vi "CALC arm angle.vi"() -> ()   [LabVIEW 2020]
uses:
  Robot Global Data.vi
panel:
  out "angle of arm pin to link pin":dbl
  out "length of arm pin to link":dbl
  in  "arm distance from center":dbl
  in  "adjust for PITCH?":bool=TRUE
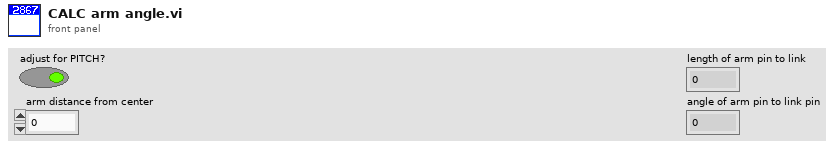
[diagram p1: front panel]
types:
  T1 = cluster{"gear ratio":cluster{"value":dbl, "descr":string}, "screw tpi":cluster{"value":dbl, "descr":string}, "shoulder AG":cluster{"value":dbl, "descr":string}, "shoulder to CTR":cluster{"value":dbl, "descr":string}, "shoulder to screw 0":cluster{"value":dbl, "descr":string}, "screw shuttle AG":cluster{"value":dbl, "descr":string}, "screw length":cluster{"value":dbl, "descr":string}, "screw to full front":cluster{"value":dbl, "descr":string}, "screw link":cluster{"value":dbl, "descr":string}, "lower arm length":cluster{"value":dbl, "descr":string}, "arm top":cluster{"value":dbl, "descr":string}, "shoulder to pin link Y":cluster{"value":dbl, "descr":string}, "shoulder to pin link X":cluster{"value":dbl, "descr":string}, "hook ht":cluster{"value":dbl, "descr":string}, "hook clear":cluster{"value":dbl, "descr":string}}
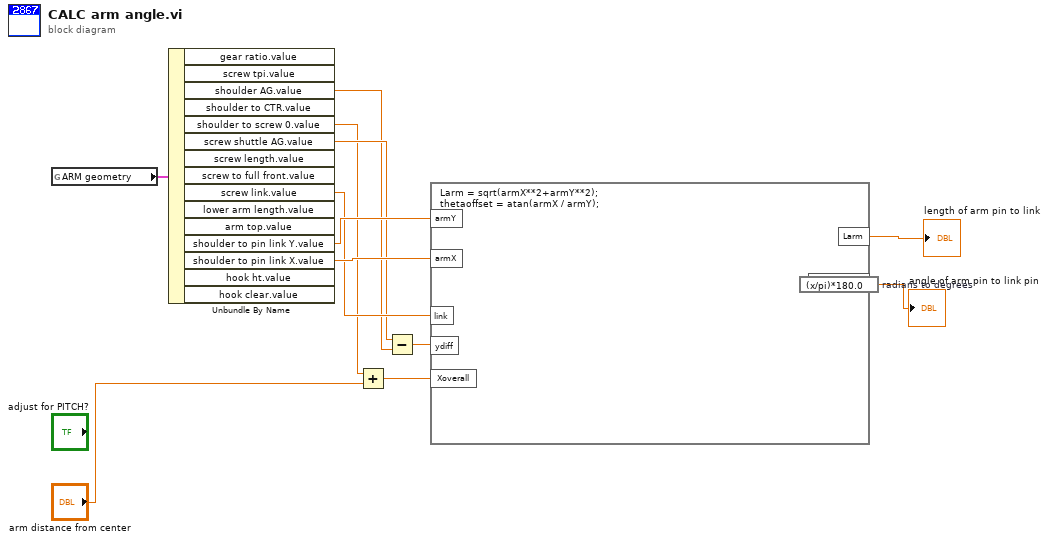
[diagram p0: block diagram]
diagram:
  n1 = global read "Robot Global Data.vi" "ARM geometry"() -> (w13:T1)
  n2 = Unbundle By Name(w13) -> ("shoulder AG.value"=w4:dbl, "shoulder to screw 0.value"=w1:dbl, "screw shuttle AG.value"=w5:dbl, "screw link.value"=w7:dbl, "shoulder to pin link Y.value"=w12:dbl, "shoulder to pin link X.value"=w11:dbl)  [unwired: 9 out]
  n3 = Add(x=w1, y="arm distance from center") -> (x+y=w3:dbl)
  n4 = Subtract(x=w5, y=w4) -> (x-y=w6:dbl)
  n5 = formula code="Larm = sqrt(armX**2+armY**2);\nthetaoffset = atan(armX / armY);"("armY"=w12, "armX"=w11, "link"=w7, "ydiff"=w6, "Xoverall"=w3) -> ("Larm"=→"length of arm pin to link":dbl, "thetaoffset"=w9:dbl)
  n6 = expression code="(x/pi)*180.0" "radians to degrees"(w9) -> (→"angle of arm pin to link pin":dbl)
